vi "main_gauge_polarisator_energy_scale.vi"() -> ()   [LabVIEW 2009]
uses:
  <vilib>/Utility/file.llb/Write To Spreadsheet File (DBL).vi
panel:
  out "Powermeter":refnum<visa-resource-name>
  in  "Anschluss von Powermeter":string="ASRL1::INSTR"
  in  "SN von Rotationsbühne":i32=83831982
  in  "MG17Motor":refnum<k7>(container)
  out "XY-Graph":cluster{dbl, dbl}[](graph)
  in  "L/2 max. [°]":dbl=180.0
  in  "L/2 min. [°]":sgl
  out "L/2 Schrittweite [°]":sgl
  out "# Messschritte":i32
  out "Messschritt":i32
  out "Vektor L/2 Wellenplatte":dbl[](array[numeric])
  out "Vektor Polarisator":dbl[](array[numeric])
  out "Polarisatorschrittweite [°]":dbl
  in  "Start Messung":bool
  in  "stop":bool
  out "Energie (iK) [W]":dbl[][](array[numeric])
  out "Energie (vK) [W]":dbl[][](array[numeric])
  in  "Polarisator min. [°]":dbl
  in  "Polarisator max. [°]":dbl=90.0
  out "Leistung [W]":dbl
  in  "Messungen/Messschritt":i32=10
  in  "# Schritte L/2 Wellenplatte":i32=36
  in  "# Schritte Polarisator":i32=9
  out "Polarisator [°]":dbl
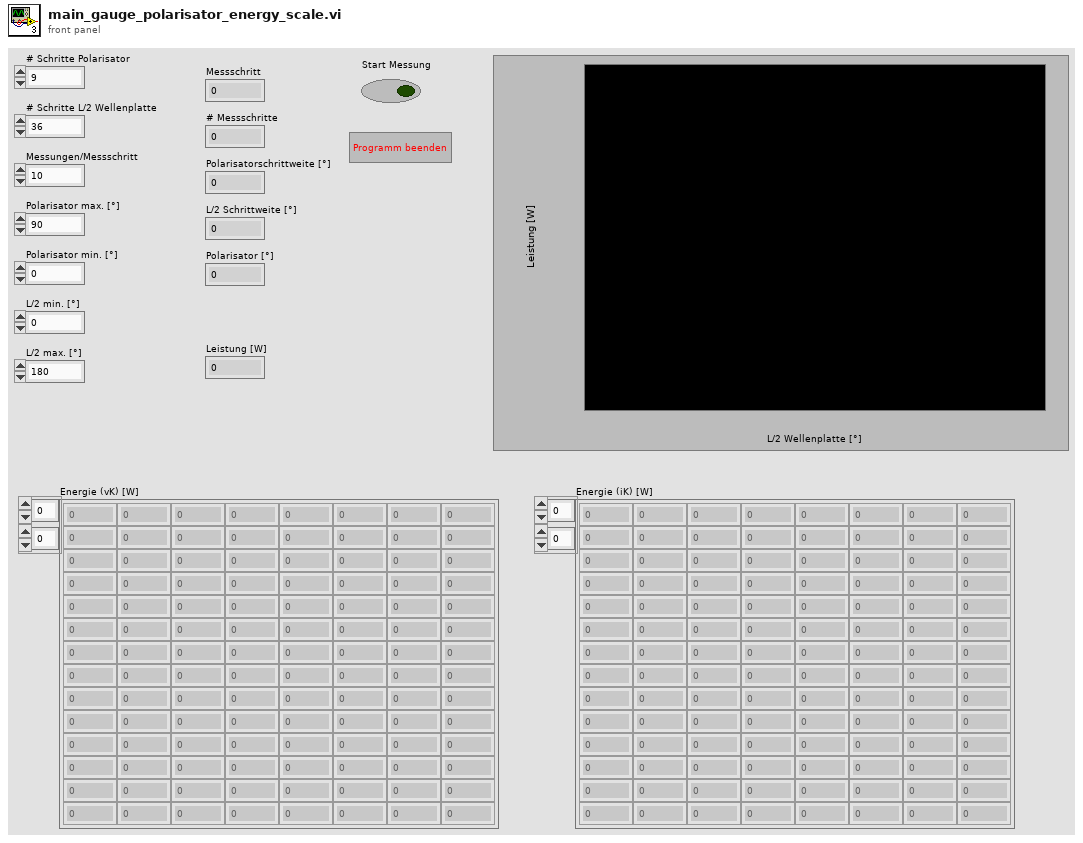
[diagram p1: front panel]
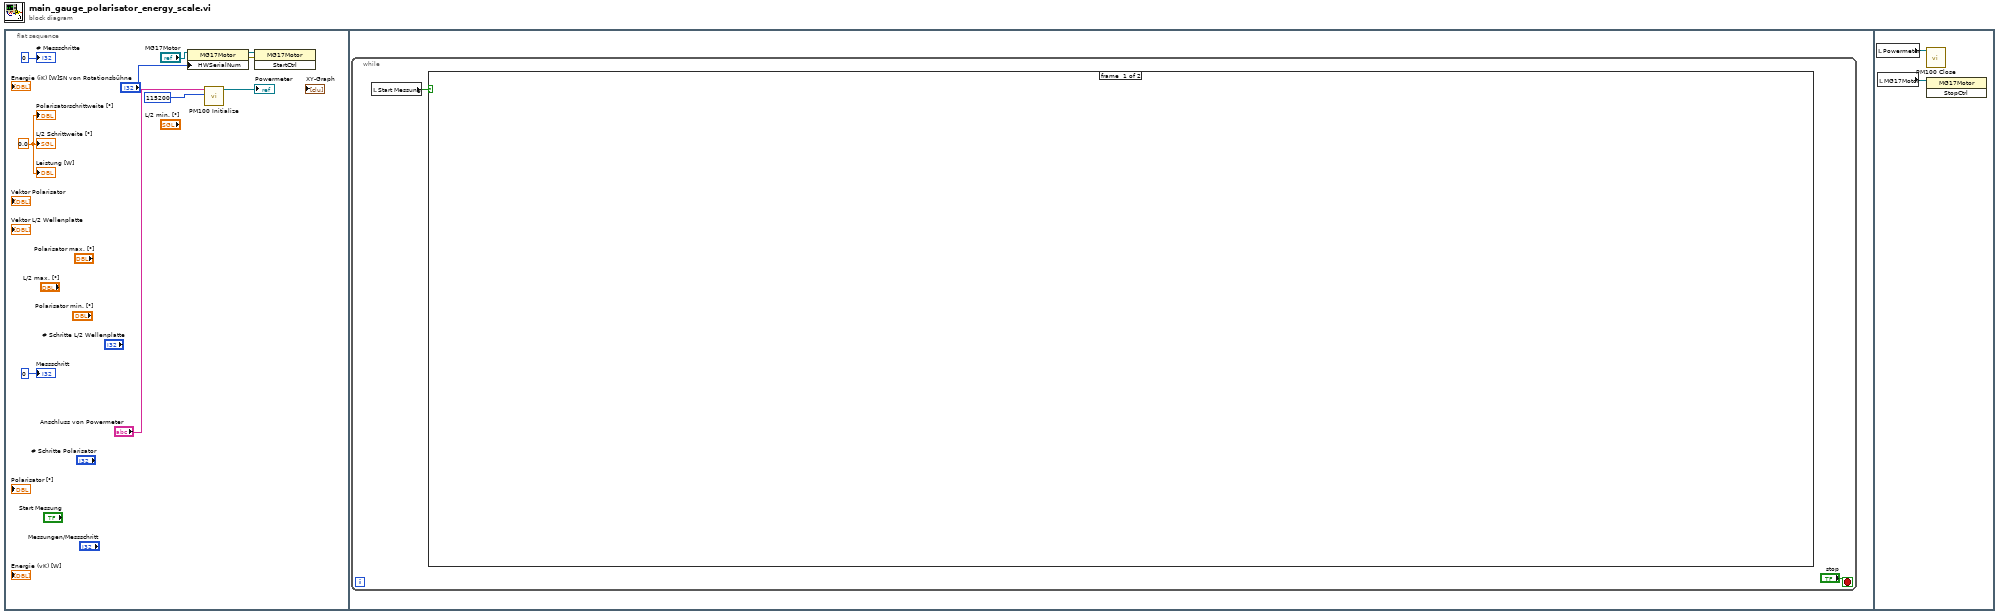
[diagram p0: block diagram]
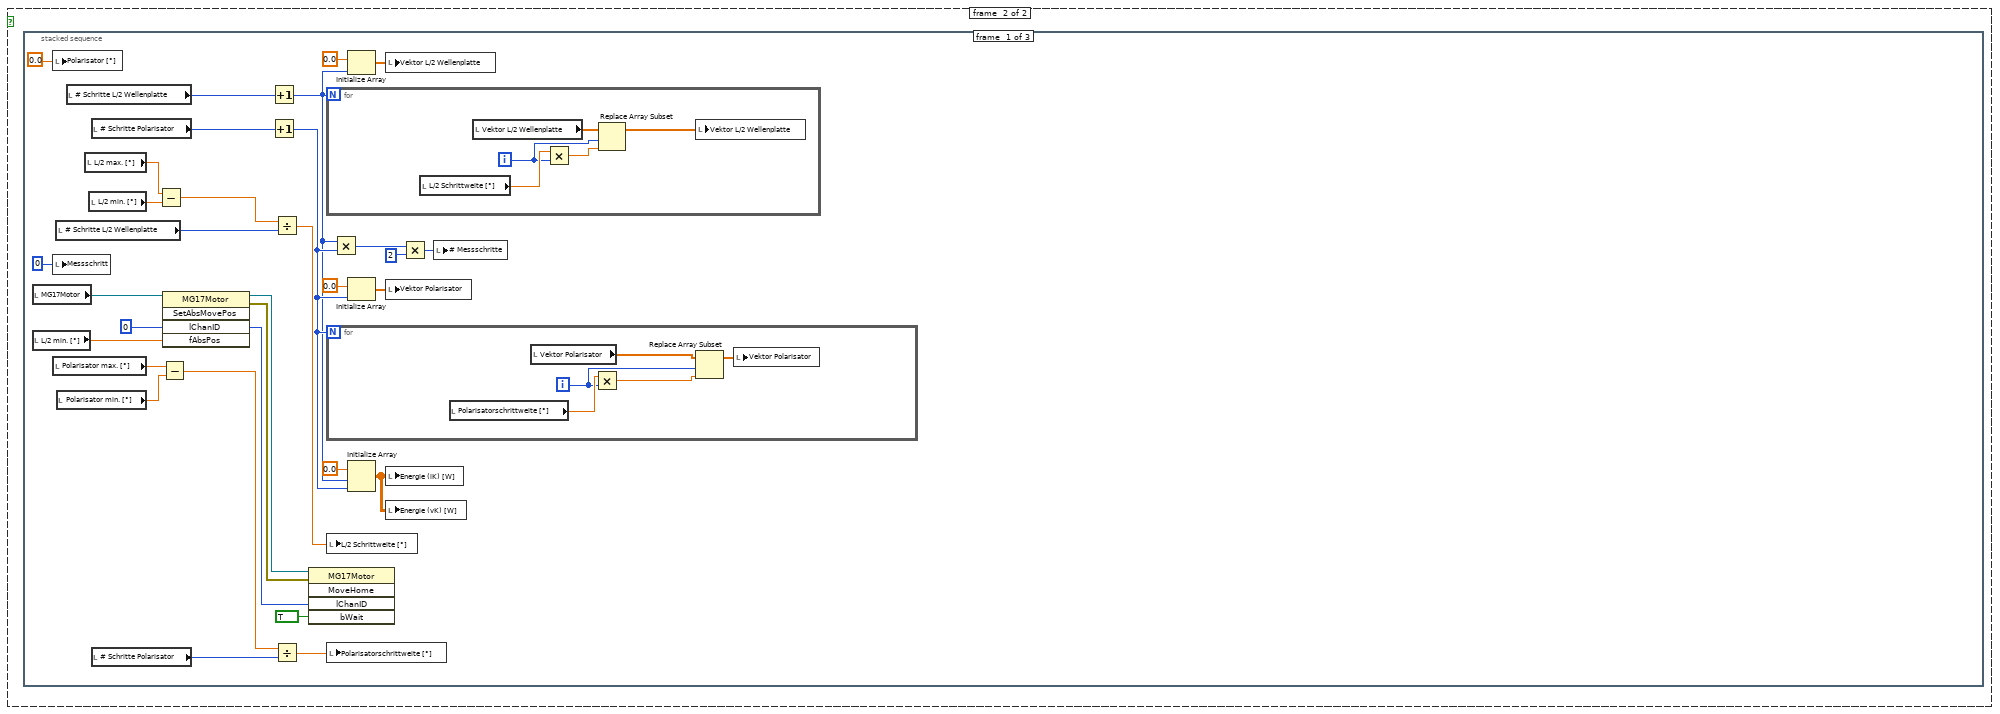
[diagram p2: hidden frame]
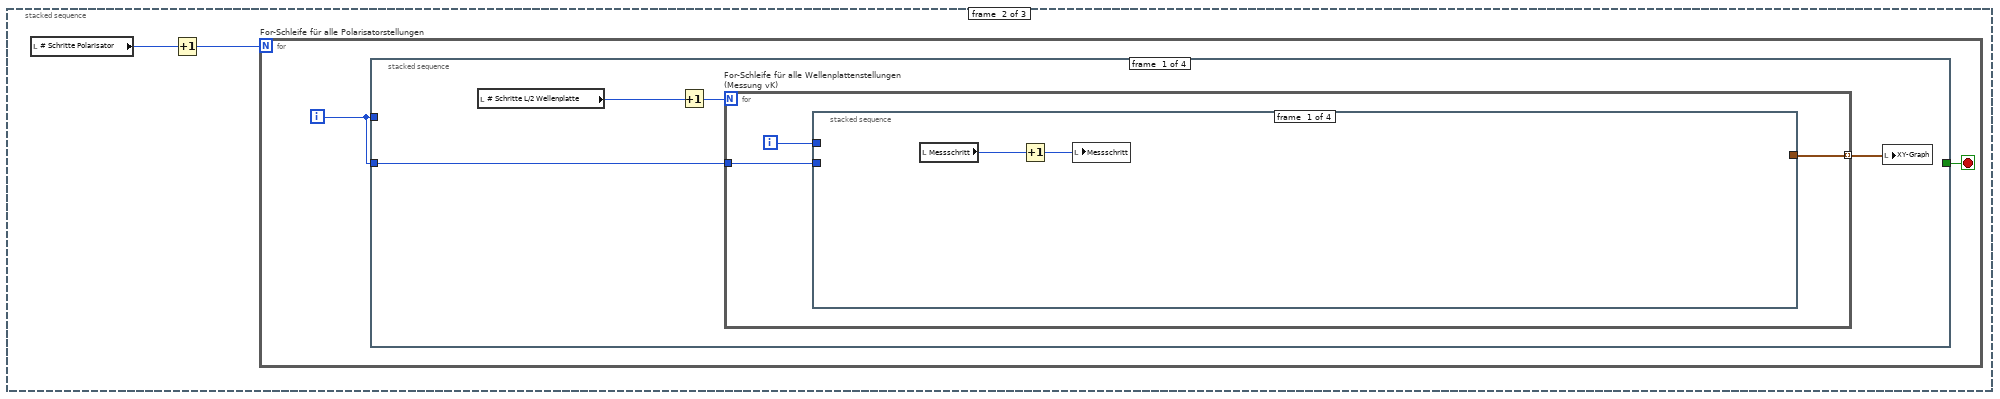
[diagram p3: hidden frame]
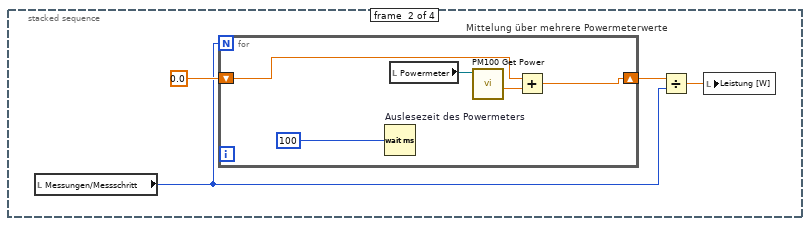
[diagram p4: hidden frame]
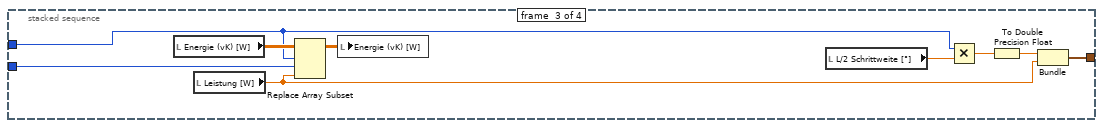
[diagram p5: hidden frame]
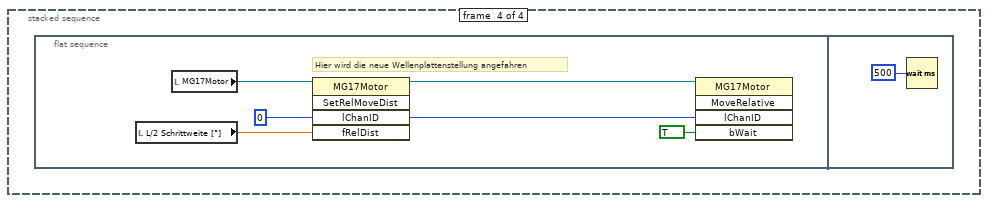
[diagram p6: hidden frame]
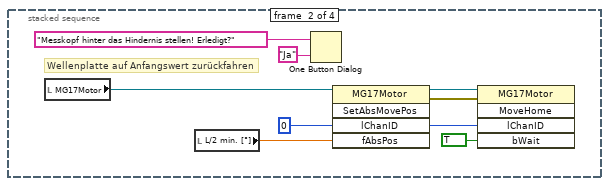
[diagram p7: hidden frame]
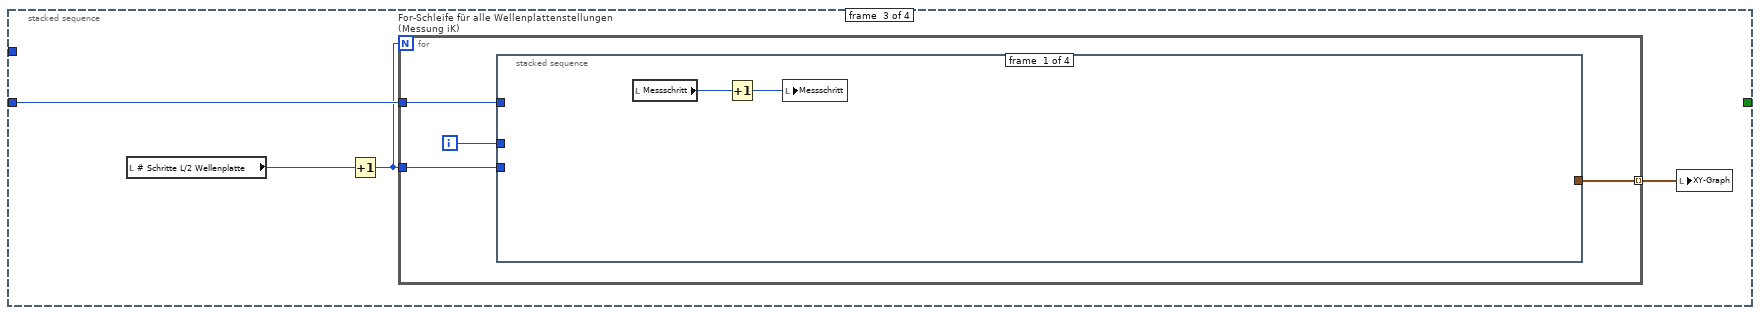
[diagram p8: hidden frame]
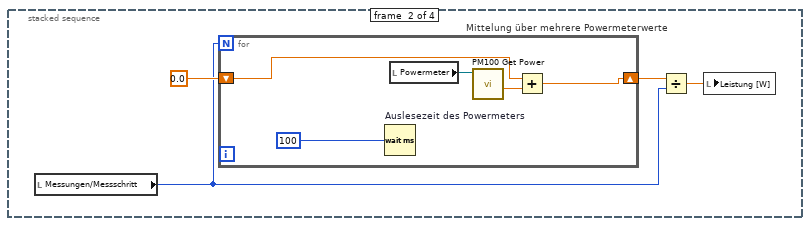
[diagram p9: hidden frame]
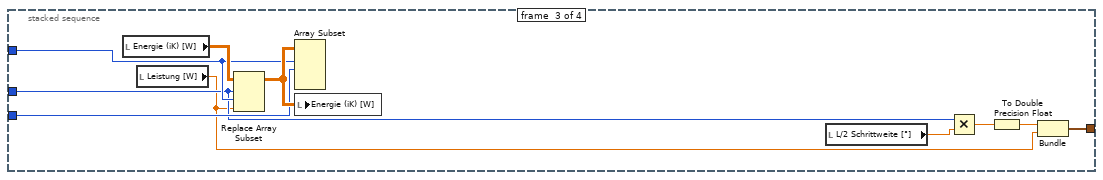
[diagram p10: hidden frame]
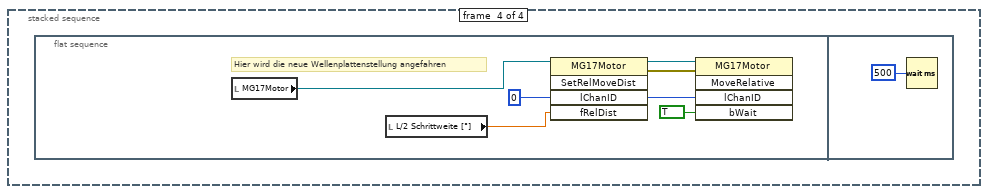
[diagram p11: hidden frame]
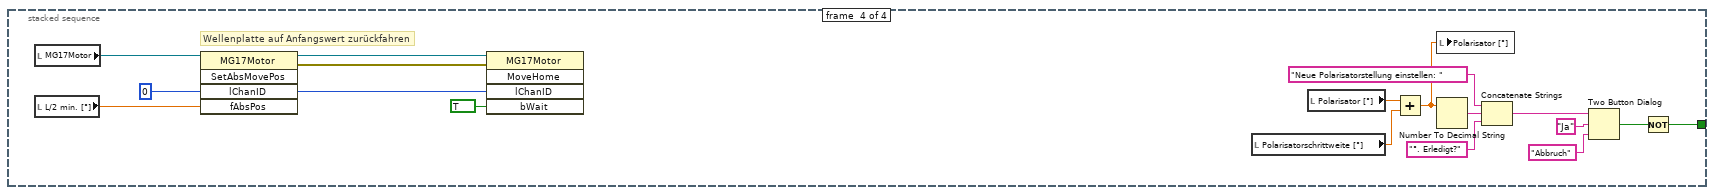
[diagram p12: hidden frame]
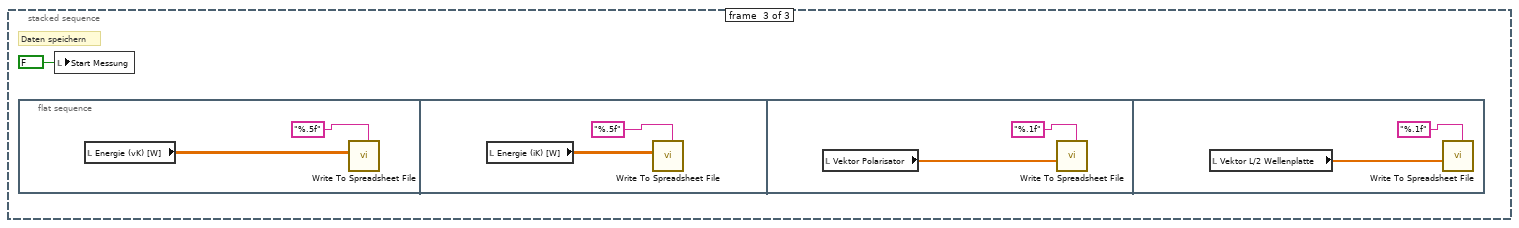
[diagram p13: hidden frame]
diagram:
  n1 = flat-sequence {
    frame #0 {
      w8 = 0.0 ("Leistung [W]")
      n2 = property class="MG17Motor"(reference="MG17Motor", "HWSerialNum"="SN von Rotationsbühne") -> (reference out=w5:refnum<k7>, error out=w4:errorcluster)  [unwired: 1 in]
      n3 = call <userlib>:"PM100 Initialize.vi"("baudrate"=115200, "resource name"="Anschluss von Powermeter") -> ("instrument handle out"=→"Powermeter":refnum<visa-resource-name>)  [unwired: 7 in, 2 out]
      n4 = invoke class="MG17Motor" method="StartCtrl"(reference=w5, error in=w4) -> ()  [unwired: 1 in, 3 out]
      "Leistung [W]" <- w8
      "Polarisatorschrittweite [°]" <- w8
      "Messschritt" <- 0 ("Messschritt")
      "# Messschritte" <- 0 ("# Messschritte")
      "L/2 Schrittweite [°]" <- w8
    }
    frame #1 {
      n5 = while {
        stop <- "stop" stop-if-true
        n6 = local read "Start Messung"() -> (w11:bool)
        n7 = case shown="True" w11 {
          frame #0 {
          }
          frame #1 {
            n8 = stacked-sequence {
              frame #0 {
                n9 = local read "MG17Motor"() -> (w15:refnum<k7>)
                n10 = local read "L/2 min. [°]"() -> (w18:sgl)
                n11 = local write "Polarisator [°]"(0.0 ("Polarisator [°]")) -> ()
                n12 = local write "Messschritt"(0 ("Messschritt 2")) -> ()
                n13 = local read "Polarisator max. [°]"() -> (w39:dbl)
                n14 = local read "# Schritte L/2 Wellenplatte"() -> (w23:i32)
                n15 = local read "Polarisator min. [°]"() -> (w40:dbl)
                n16 = local read "# Schritte L/2 Wellenplatte"() -> (w32:i32)
                n17 = local read "L/2 max. [°]"() -> (w26:dbl)
                n18 = local read "L/2 min. [°]"() -> (w25:sgl)
                n19 = local read "# Schritte Polarisator"() -> (w31:i32)
                n20 = local read "# Schritte Polarisator"() -> (w42:i32)
                n21 = Subtract(x=w26, y=w25) -> (x-y=w24:dbl)
                n22 = Subtract(x=w39, y=w40) -> (x-y=w41:dbl)
                n23 = invoke class="MG17Motor" method="SetAbsMovePos"(reference=w15, "lChanID"=0, "fAbsPos"=w18) -> (reference out=w20:refnum<k7>, error out=w19:errorcluster, "lChanID"=w16:i32)  [unwired: 2 in, 2 out]
                n24 = Increment(x=w32) -> (x+1=w13:i32)
                n25 = Increment(x=w31) -> (x+1=w21:i32)
                n26 = Divide(x=w24, y=w23) -> (x/y=w22:dbl)
                n27 = Divide(x=w41, y=w42) -> (x/y=w43:dbl)
                n28 = invoke class="MG17Motor" method="MoveHome"(reference=w20, error in=w19, "lChanID"=w16, "bWait"=TRUE) -> ()  [unwired: 1 in, 5 out]
                n29 = for {
                  N: w13 -> [_]
                  i -> [w51]
                  n30 = local read "L/2 Schrittweite [°]"() -> (w54:sgl)
                  n31 = local read "Vektor L/2 Wellenplatte"() -> (w53:dbl[])
                  n32 = Multiply(x=w54, y=w51) -> (x*y=w50:sgl)
                  n33 = Replace Array Subset(array=w53, new element=w50, index=w51) -> (w52:dbl[])
                  n34 = local write "Vektor L/2 Wellenplatte"(w52) -> ()
                }
                n35 = for {
                  N: w21 -> [_]
                  i -> [w46]
                  n36 = local read "Polarisatorschrittweite [°]"() -> (w49:dbl)
                  n37 = local read "Vektor Polarisator"() -> (w48:dbl[])
                  n38 = Multiply(x=w49, y=w46) -> (x*y=w45:dbl)
                  n39 = Replace Array Subset(array=w48, new element=w45, index=w46) -> (w47:dbl[])
                  n40 = local write "Vektor Polarisator"(w47) -> ()
                }
                n41 = local write "L/2 Schrittweite [°]"(w22) -> ()
                n42 = local write "Polarisatorschrittweite [°]"(w43) -> ()
                n43 = Multiply(x=w13, y=w21) -> (x*y=w36:i32)
                n44 = Initialize Array(0.0 ("element"), w13) -> (w28:dbl[])
                n45 = Initialize Array(0.0 ("element"), w21) -> (w27:dbl[])
                n46 = Initialize Array(0.0 ("element"), w13, w21) -> (w34:dbl[][])
                n47 = local write "Vektor L/2 Wellenplatte"(w28) -> ()
                n48 = local write "Vektor Polarisator"(w27) -> ()
                n49 = local write "Energie (iK) [W]"(w34) -> ()
                n50 = local write "Energie (vK) [W]"(w34) -> ()
                n51 = Multiply(x=w36, y=2) -> (x*y=w37:i32)
                n52 = local write "# Messschritte"(w37) -> ()
              }
              frame #1 {
                n53 = local read "# Schritte Polarisator"() -> (w56:i32)
                n54 = Increment(x=w56) -> (x+1=w55:i32)
                n55 = for "For-Schleife für alle Polarisatorstellungen" {
                  N: w55 -> [_]
                  i -> [w58]
                  stop <- w57 stop-if-true
                  n56 = stacked-sequence {
                    tunnel: w58 -> [w62 _ w104 _]
                    tunnel: w58 -> [_ _ _ _]
                    tunnel: [_ _ _ w146] -> w57
                    frame #0 {
                      n57 = local read "# Schritte L/2 Wellenplatte"() -> (w61:i32)
                      n58 = Increment(x=w61) -> (x+1=w60:i32)
                      n59 = for "For-Schleife für alle Wellenplattenstellungen (Messung vK)" {
                        N: w60 -> [_]
                        tunnel: w62 -> [w64]
                        tunnel: [w63] -> w59 mode=indexing
                        i -> [w65]
                        n60 = stacked-sequence {
                          tunnel: w65 -> [_ _ w78 _]
                          tunnel: w64 -> [_ _ w83 _]
                          tunnel: [_ _ w77 _] -> w63
                          frame #0 {
                            n61 = local read "Messschritt"() -> (w66:i32)
                            n62 = Increment(x=w66) -> (x+1=w67:i32)
                            n63 = local write "Messschritt"(w67) -> ()
                          }
                          frame #1 {
                            n64 = local read "Messungen/Messschritt"() -> (w68:i32)
                            n65 = for "Mittelung über mehrere Powermeterwerte" {
                              N: w68 -> [_]
                              shift-right: [w75] -> w70
                              shift-left: 0.0 -> [w76]
                              n66 = Wait (ms) "Auslesezeit des Powermeters"(milliseconds to wait=u32 100 ("Zu wartende ms")) -> ()  [unwired: 1 out]
                              n67 = local read "Powermeter"() -> (w72:refnum<visa-resource-name>)
                              n68 = call <userlib>:"PM100 Get Power.vi"("instrument handle"=w72) -> ("power"=w74:dbl)  [unwired: 7 in, 3 out]
                              n69 = Add(x=w76, y=w74) -> (x+y=w75:dbl)
                            }
                            n70 = Divide(x=w70, y=w68) -> (x/y=w69:dbl)
                            n71 = local write "Leistung [W]"(w69) -> ()
                          }
                          frame #2 {
                            n72 = local read "Energie (vK) [W]"() -> (w85:dbl[][])
                            n73 = local read "Leistung [W]"() -> (w79:dbl)
                            n74 = Replace Array Subset(array=w85, new element=w79, index (row)=w78, index (col)=w83) -> (w84:dbl[][])
                            n75 = local write "Energie (vK) [W]"(w84) -> ()
                            n76 = local read "L/2 Schrittweite [°]"() -> (w82:sgl)
                            n77 = Multiply(x=w78, y=w82) -> (x*y=w81:sgl)
                            n78 = To Double Precision Float(number=w81) -> (double precision float=w80:dbl)
                            n79 = Bundle(w80, "Leistung [W]"=w79) -> (w77:cluster{dbl, "Leistung [W]":dbl})  [unwired: 1 in]
                          }
                          frame #3 {
                            n80 = flat-sequence {
                              frame #0 {
                                # "Hier wird die neue Wellenplattenstellung angefahren"
                                n81 = local read "L/2 Schrittweite [°]"() -> (w90:sgl)
                                n82 = local read "MG17Motor"() -> (w86:refnum<k7>)
                                n83 = invoke class="MG17Motor" method="SetRelMoveDist"(reference=w86, "lChanID"=0, "fRelDist"=w90) -> (reference out=w88:refnum<k7>, "lChanID"=w89:i32)  [unwired: 2 in, 3 out]
                                n84 = invoke class="MG17Motor" method="MoveRelative"(reference=w88, "lChanID"=w89, "bWait"=TRUE) -> ()  [unwired: 2 in, 5 out]
                              }
                              frame #1 {
                                n85 = Wait (ms)(milliseconds to wait=u32 500 ("Zu wartende ms")) -> ()  [unwired: 1 out]
                              }
                            }
                          }
                        }
                      }
                      n86 = local write "XY-Graph"(w59) -> ()
                    }
                    frame #1 {
                      # "Wellenplatte auf Anfangswert zurückfahren"
                      n87 = local read "MG17Motor"() -> (w95:refnum<k7>)
                      n88 = local read "L/2 min. [°]"() -> (w99:sgl)
                      n89 = One Button Dialog(message="Messkopf hinter das Hindernis stellen! Erledigt?", button name ("OK")="Ja") -> ()  [unwired: 1 out]
                      n90 = invoke class="MG17Motor" method="SetAbsMovePos"(reference=w95, "lChanID"=0, "fAbsPos"=w99) -> (reference out=w101:refnum<k7>, error out=w100:errorcluster, "lChanID"=w97:i32)  [unwired: 2 in, 2 out]
                      n91 = invoke class="MG17Motor" method="MoveHome"(reference=w101, error in=w100, "lChanID"=w97, "bWait"=TRUE) -> ()  [unwired: 1 in, 5 out]
                    }
                    frame #2 {
                      n92 = local read "# Schritte L/2 Wellenplatte"() -> (w105:i32)
                      n93 = Increment(x=w105) -> (x+1=w103:i32)
                      n94 = for "For-Schleife für alle Wellenplattenstellungen (Messung iK)" {
                        N: w103 -> [_]
                        tunnel: w104 -> [w109]
                        tunnel: w103 -> [w107]
                        tunnel: [w106] -> w102 mode=indexing
                        i -> [w108]
                        n95 = stacked-sequence {
                          tunnel: w108 -> [_ _ w126 _]
                          tunnel: w109 -> [_ _ w128 _]
                          tunnel: w107 -> [_ _ w127 _]
                          tunnel: [_ _ w121 _] -> w106
                          frame #0 {
                            n96 = local read "Messschritt"() -> (w111:i32)
                            n97 = Increment(x=w111) -> (x+1=w110:i32)
                            n98 = local write "Messschritt"(w110) -> ()
                          }
                          frame #1 {
                            n99 = local read "Messungen/Messschritt"() -> (w112:i32)
                            n100 = for "Mittelung über mehrere Powermeterwerte" {
                              N: w112 -> [_]
                              shift-right: [w119] -> w114
                              shift-left: 0.0 -> [w120]
                              n101 = Wait (ms) "Auslesezeit des Powermeters"(milliseconds to wait=u32 100 ("Zu wartende ms")) -> ()  [unwired: 1 out]
                              n102 = local read "Powermeter"() -> (w116:refnum<visa-resource-name>)
                              n103 = call <userlib>:"PM100 Get Power.vi"("instrument handle"=w116) -> ("power"=w118:dbl)  [unwired: 7 in, 3 out]
                              n104 = Add(x=w120, y=w118) -> (x+y=w119:dbl)
                            }
                            n105 = Divide(x=w114, y=w112) -> (x/y=w113:dbl)
                            n106 = local write "Leistung [W]"(w113) -> ()
                          }
                          frame #2 {
                            n107 = local read "Energie (iK) [W]"() -> (w130:dbl[][])
                            n108 = local read "Leistung [W]"() -> (w124:dbl)
                            n109 = Replace Array Subset(array=w130, new element=w124, index (row)=w126, index (col)=w128) -> (w129:dbl[][])
                            n110 = Array Subset(array=w129, index (row)=w128, length (row)=w127) -> ()  [unwired: 2 in, 1 out]
                            n111 = local write "Energie (iK) [W]"(w129) -> ()
                            n112 = local read "L/2 Schrittweite [°]"() -> (w125:sgl)
                            n113 = Multiply(x=w126, y=w125) -> (x*y=w123:sgl)
                            n114 = To Double Precision Float(number=w123) -> (double precision float=w122:dbl)
                            n115 = Bundle(w122, "Leistung [W]"=w124) -> (w121:cluster{dbl, "Leistung [W]":dbl})  [unwired: 1 in]
                          }
                          frame #3 {
                            n116 = flat-sequence {
                              frame #0 {
                                # "Hier wird die neue Wellenplattenstellung angefahren"
                                n117 = local read "MG17Motor"() -> (w132:refnum<k7>)
                                n118 = local read "L/2 Schrittweite [°]"() -> (w136:sgl)
                                n119 = invoke class="MG17Motor" method="SetRelMoveDist"(reference=w132, "lChanID"=0, "fRelDist"=w136) -> (reference out=w134:refnum<k7>, error out=w133:errorcluster, "lChanID"=w135:i32)  [unwired: 2 in, 2 out]
                                n120 = invoke class="MG17Motor" method="MoveRelative"(reference=w134, error in=w133, "lChanID"=w135, "bWait"=TRUE) -> ()  [unwired: 1 in, 5 out]
                              }
                              frame #1 {
                                n121 = Wait (ms)(milliseconds to wait=u32 500 ("Zu wartende ms")) -> ()  [unwired: 1 out]
                              }
                            }
                          }
                        }
                      }
                      n122 = local write "XY-Graph"(w102) -> ()
                    }
                    frame #3 {
                      # "Wellenplatte auf Anfangswert zurückfahren"
                      n123 = local read "MG17Motor"() -> (w139:refnum<k7>)
                      n124 = local read "L/2 min. [°]"() -> (w143:sgl)
                      n125 = invoke class="MG17Motor" method="SetAbsMovePos"(reference=w139, "lChanID"=0, "fAbsPos"=w143) -> (reference out=w145:refnum<k7>, error out=w144:errorcluster, "lChanID"=w141:i32)  [unwired: 2 in, 2 out]
                      n126 = invoke class="MG17Motor" method="MoveHome"(reference=w145, error in=w144, "lChanID"=w141, "bWait"=TRUE) -> ()  [unwired: 1 in, 5 out]
                      n127 = local read "Polarisatorschrittweite [°]"() -> (w155:dbl)
                      n128 = local read "Polarisator [°]"() -> (w156:dbl)
                      n129 = Add(x=w156, y=w155) -> (x+y=w147:dbl)
                      n130 = local write "Polarisator [°]"(w147) -> ()
                      n131 = Number To Decimal String(number=w147) -> (decimal integer string=w153:string)  [unwired: 1 in]
                      n132 = Concatenate Strings("Neue Polarisatorstellung einstellen: " ("message"), w153, "°. Erledigt?" ("string")) -> (w151:string)
                      n133 = Two Button Dialog(message=w151, 1:"Abbruch" ("F button name (\"Cancel\")"), 2:"Ja" ("button name (\"OK\")")) -> (T button?=w148:bool)
                      n134 = Not(x=w148) -> (.not. x?=w146:bool)
                    }
                  }
                }
              }
              frame #2 {
                # "Daten speichern"
                n135 = flat-sequence {
                  frame #0 {
                    n136 = local read "Energie (vK) [W]"() -> (w158:dbl[][])
                    n137 = call-poly <vilib>:"Write To Spreadsheet File.vi"("format (%.3f)"="%.5f", "2D data"=w158) -> ()  [unwired: 6 in, 1 out]
                  }
                  frame #1 {
                    n138 = local read "Energie (iK) [W]"() -> (w160:dbl[][])
                    n139 = call-poly <vilib>:"Write To Spreadsheet File.vi"("format (%.3f)"="%.5f", "2D data"=w160) -> ()  [unwired: 6 in, 1 out]
                  }
                  frame #2 {
                    n140 = local read "Vektor Polarisator"() -> (w162:dbl[])
                    n141 = call-poly <vilib>:"Write To Spreadsheet File.vi"("format (%.3f)"="%.1f", "1D data"=w162) -> ()  [unwired: 6 in, 1 out]
                  }
                  frame #3 {
                    n142 = local read "Vektor L/2 Wellenplatte"() -> (w164:dbl[])
                    n143 = call-poly <vilib>:"Write To Spreadsheet File.vi"("format (%.3f)"="%.1f", "1D data"=w164) -> ()  [unwired: 6 in, 1 out]
                  }
                }
                n144 = local write "Start Messung"(FALSE ("Start Messung")) -> ()
              }
            }
          }
        }
      }
    }
    frame #2 {
      n145 = local read "Powermeter"() -> (w166:refnum<visa-resource-name>)
      n146 = local read "MG17Motor"() -> (w167:refnum<k7>)
      n147 = call <userlib>:"PM100 Close.vi"("instrument handle"=w166) -> ()  [unwired: 9 in, 2 out]
      n148 = invoke class="MG17Motor" method="StopCtrl"(reference=w167) -> ()  [unwired: 2 in, 3 out]
    }
  }
